vi "Sine ramps pattern.vi"(10 "Waveform parameters 2":T1={"Start magnitude"=1000.0, "Magnitude increment"=1000.0, "Number of pulses"=8, "Ramp length"=32, "Top  length"=480, "Threshold "=3000, "Processing delay"=240, "Stop after"=1, "Detector window"=480} {"Detector window" format="%dpts"; "Stop after" format="%d sweep(s)"}) -> (2 "Waveform":dbl[](array[numeric]), 3 "Waveform parameters out":T1={"Start magnitude"=0.0, "Magnitude increment"=0.0, "Number of pulses"=0, "Ramp length"=0, "Top  length"=0, "Threshold "=3000, "Processing delay"=240, "Stop after"=1, "Detector window"=480} {"Detector window" format="%dpts"; "Stop after" format="%d sweep(s)"})   [LabVIEW 2019]
uses:
  Waveform parameters.ctl
panel:
  out "I-V waveform":dbl[](graph)
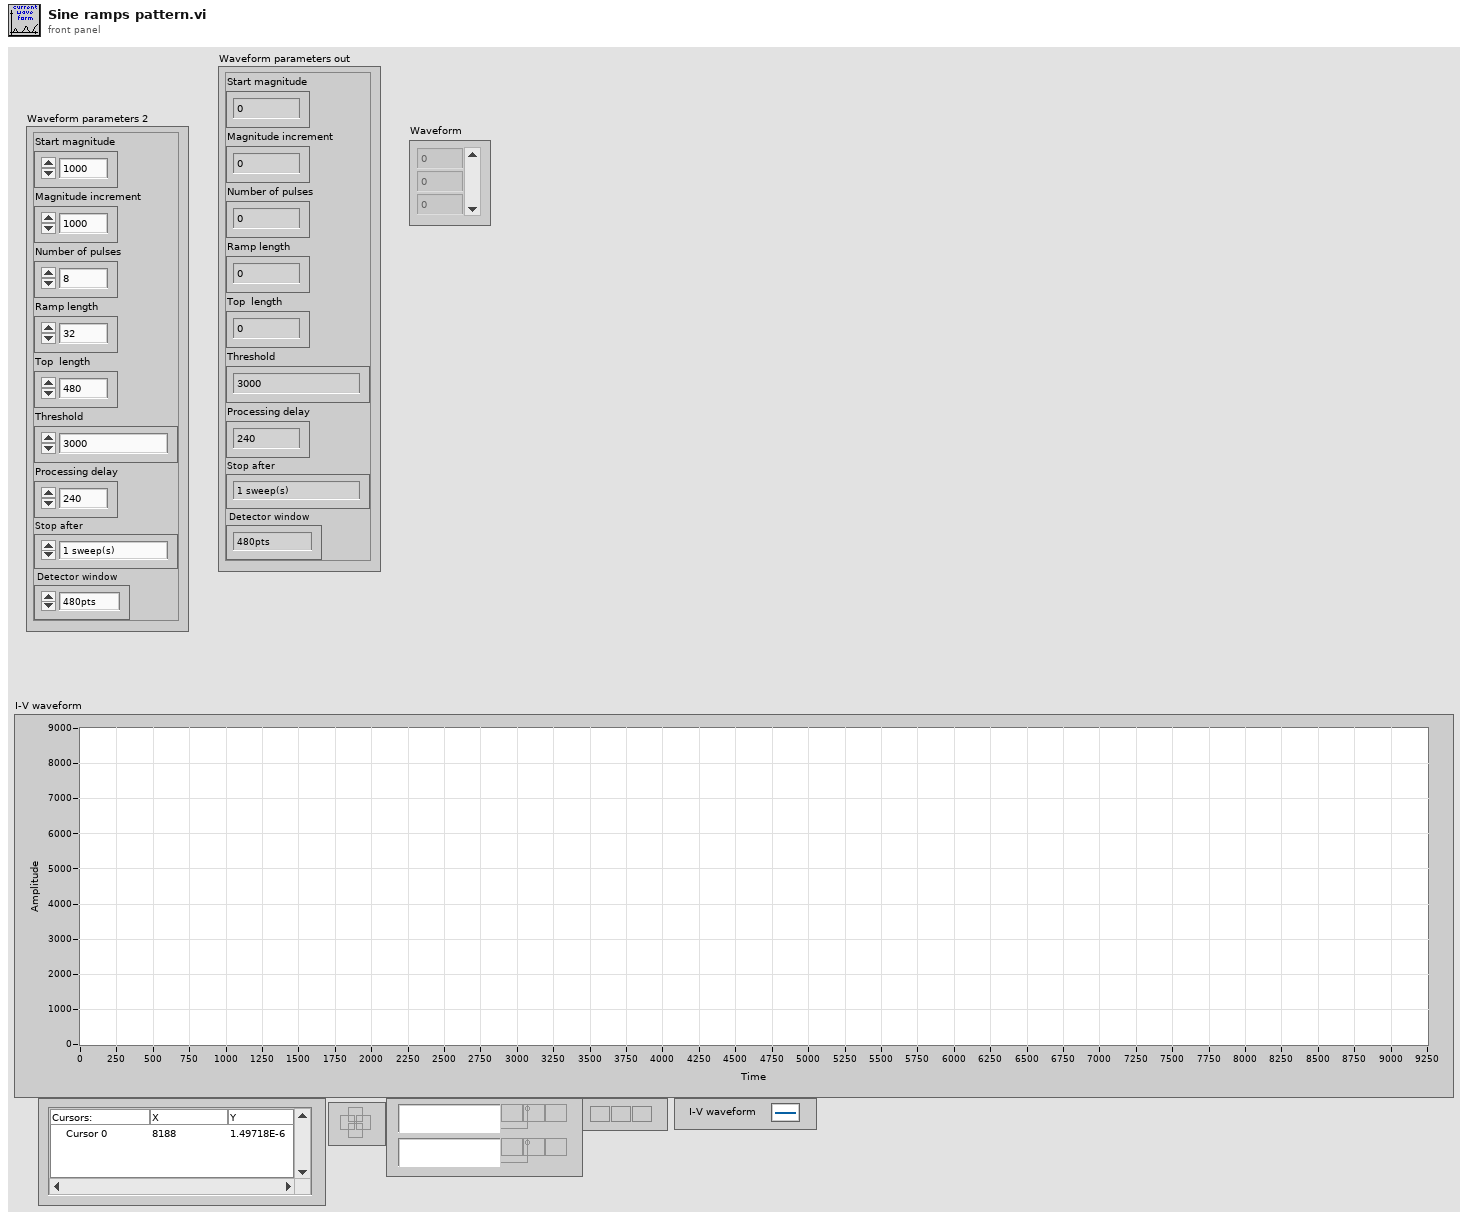
[diagram p1: front panel]
types:
  T1 = typedef "Waveform parameters.ctl" = cluster{"Start magnitude":dbl, "Magnitude increment":dbl, "Number of pulses":i32, "Ramp length":i32, "Top  length":i32, "Threshold ":i32, "Processing delay":u16, "Stop after":u16, "Detector window":i32}
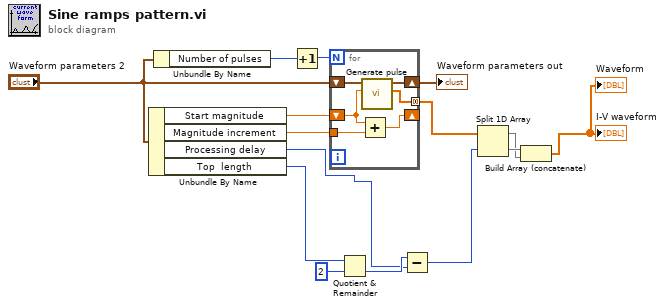
[diagram p0: block diagram]
diagram:
  n1 = Unbundle By Name("Waveform parameters 2") -> ("Start magnitude"=w12:dbl, "Magnitude increment"=w11:dbl, "Processing delay"=w1:u16, "Top  length"=w5:i32)
  n2 = Unbundle By Name("Waveform parameters 2") -> ("Number of pulses"=w14:i32)
  n3 = Increment(x=w14) -> (x+1=w10:i32)
  n4 = for {
    N: w10 -> [_]
    shift-right: [w20] -> w15
    shift-left: "Waveform parameters 2" -> [w21]
    tunnel: [w19] -> w9 mode=concatenating
    shift-right: [w16] -> _
    shift-left: w12 -> [w18]
    tunnel: w11 -> [w17]
    n5 = Add(x=w18, y=w17) -> (x+y=w16:dbl)
    n6 = call "Generate pulse.vi"("Pulse magnitude"=w18, "Waveform parameters"=w21) -> ("Data out"=w19:dbl[], "Waveform parameters out"=w20:T1)  [unwired: 8 in]
  }
  "Waveform parameters out" <- w15
  n7 = Quotient & Remainder(x=w5, y=2) -> (floor(x/y)=w2:i32)  [unwired: 1 out]
  n8 = Subtract(x=w2, y=w1) -> (x-y=w3:i32)
  n9 = Split 1D Array(array=w9, index=w3) -> (first subarray=w6:dbl[], second subarray=w7:dbl[])
  n10 = Build Array (concatenate)(w7, w6) -> (→"I-V waveform" →"Waveform":dbl[])
